vi "WASDDRIVE.vi"(9 "RIGHTIN":i8, 10 "LEFTIN":i8, 11 "KEY":i16) -> (2 "RIGHTOUT":i8, 3 "LEFTOUT":i8)   [LabVIEW 2017]
panel:
  # "This is the WASD motor control VI. It takes in key presses and outputs motor values based on those."
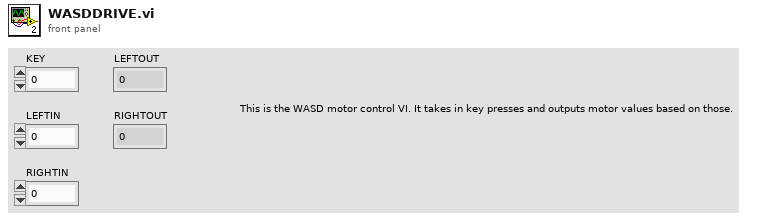
[diagram p1: front panel]
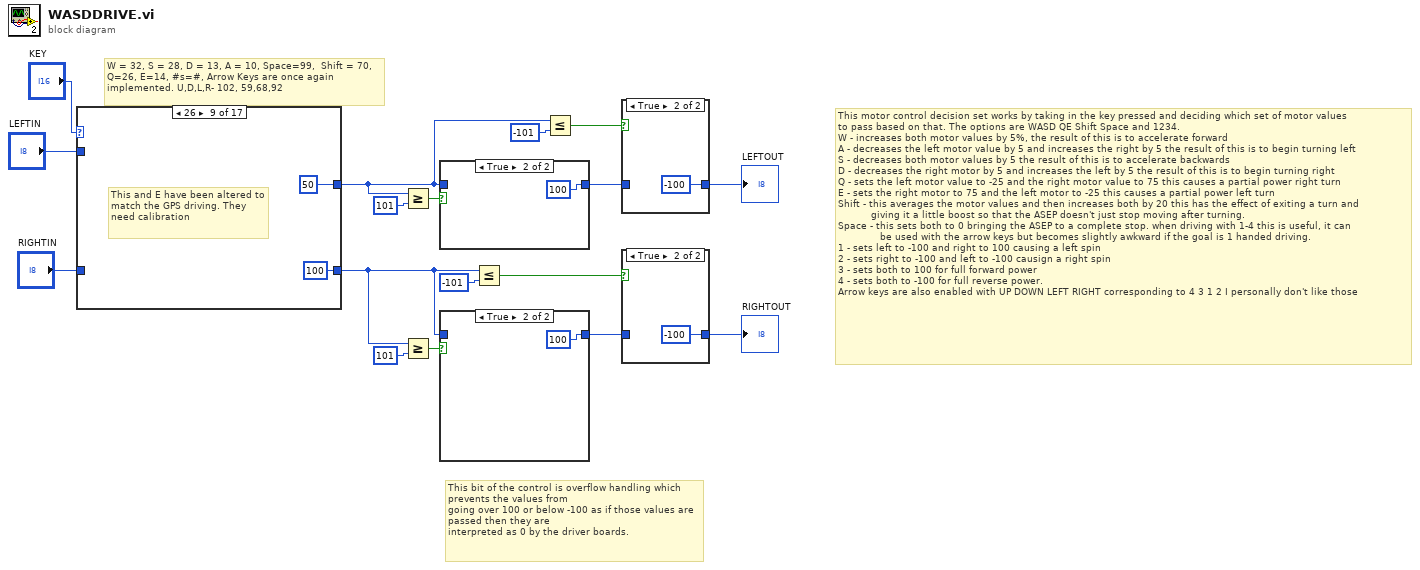
[diagram p0: block diagram]
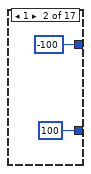
[diagram p7: hidden frame]
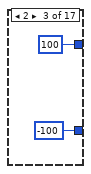
[diagram p8: hidden frame]
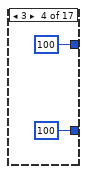
[diagram p9: hidden frame]
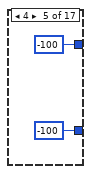
[diagram p10: hidden frame]
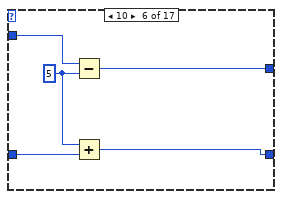
[diagram p11: hidden frame]
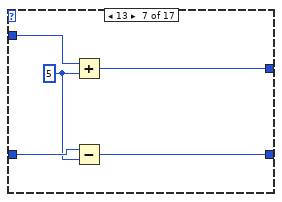
[diagram p12: hidden frame]
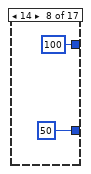
[diagram p13: hidden frame]
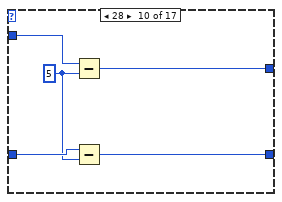
[diagram p14: hidden frame]
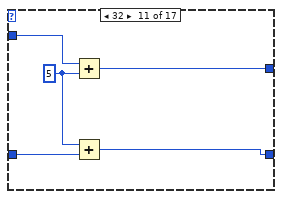
[diagram p15: hidden frame]
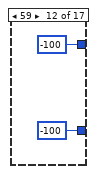
[diagram p16: hidden frame]
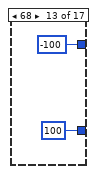
[diagram p17: hidden frame]
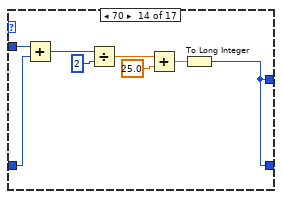
[diagram p18: hidden frame]
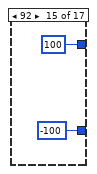
[diagram p19: hidden frame]
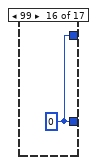
[diagram p20: hidden frame]
diagram:
  # "This bit of the control is overflow handling which prevents the values from \ngoing over 100 or below -100 as if those values are passed then they are \ninterpreted as 0 by the driver boards."
  # "This motor control decision set works by taking in the key pressed and deciding which set of motor values\nto pass based on that. The options are WASD QE Shift Space and 1234. \nW - increases both motor values by 5%, the result of this is to accelerate forward\nA - decreases the left motor value by 5 and increases the right by 5 the result of this is to begin turning left\nS - decreases both motor values by 5 the result of this is to accelerate backwards\nD - decreases the right motor by 5 and increases the left by 5 the result of this is to begin turning right\nQ - sets the left motor value to -25 and the right motor value to 75 this causes a partial power right turn\nE - sets the right motor to 75 and the left motor to -25 this causes a partial power left turn\nShift - this averages the motor values and then increases both by 20 this has the effect of exiting a turn and\n           giving it a little boost so that the ASEP doesn't just stop moving after turning. \nSpace - this sets both to 0 bringing the ASEP to a complete stop. when driving with 1-4 this is useful, it can \n              be used with the arrow keys but becomes slightly awkward if the goal is 1 handed driving. \n1 - sets left to -100 and right to 100 causing a left spin\n2 - sets right to -100 and left to -100 causign a right spin\n3 - sets both to 100 for full forward power\n4 - sets both to -100 for full reverse power.\nArrow keys are also enabled with UP DOWN LEFT RIGHT corresponding to 4 3 1 2 I personally don't like those"
  # "W = 32, S = 28, D = 13, A = 10, Space=99,  Shift = 70, Q=26, E=14, #s=#, Arrow Keys are once again implemented. U,D,L,R- 102, 59,68,92"
  n1 = case shown="26" "KEY" {
    tunnel: [w18 100 -100 100 -100 w31 w33 50 100 w43 w48 -100 100 w59 -100 w66 100] -> w14
    tunnel: [w19 -100 100 100 -100 w28 w36 100 50 w45 w47 -100 -100 w59 100 w66 100] -> w7
    tunnel: "LEFTIN" -> [w19 _ _ _ _ w29 w37 _ _ w46 w51 _ _ w63 _ _ _]
    tunnel: "RIGHTIN" -> [w18 _ _ _ _ w32 w35 _ _ w44 w49 _ _ w62 _ _ _]
    frame 0, Default {
    }
    frame 1 {
    }
    frame 2 {
    }
    frame 3 {
    }
    frame 4 {
    }
    frame 10 {
      w30 = 5
      n2 = Subtract(x=w29, y=w30) -> (x-y=w28:i32)
      n3 = Add(x=w30, y=w32) -> (x+y=w31:i32)
    }
    frame 13 {
      w34 = 5
      n4 = Add(x=w37, y=w34) -> (x+y=w36:i32)
      n5 = Subtract(x=w35, y=w34) -> (x-y=w33:i32)
    }
    frame 14 {
    }
    frame 26 {
      # "This and E have been altered to match the GPS driving. They need calibration"
    }
    frame 28 {
      w42 = 5
      n6 = Subtract(x=w46, y=w42) -> (x-y=w45:i32)
      n7 = Subtract(x=w44, y=w42) -> (x-y=w43:i32)
    }
    frame 32 {
      w50 = 5
      n8 = Add(x=w51, y=w50) -> (x+y=w47:i32)
      n9 = Add(x=w50, y=w49) -> (x+y=w48:i32)
    }
    frame 59 {
    }
    frame 68 {
    }
    frame 70 {
      n10 = Add(x=w63, y=w62) -> (x+y=w61:i8)
      n11 = Divide(x=w61, y=2) -> (x/y=w58:dbl)
      n12 = Add(x=w58, y=25.0) -> (x+y=w57:dbl)
      n13 = To Long Integer(number=w57) -> (32bit integer=w59:i32)
    }
    frame 92 {
    }
    frame 99 {
      w66 = 0
    }
    frame 102 {
    }
  }
  n14 = Greater Or Equal?(x=w7, y=101) -> (x >= y?=w6:bool)
  n15 = Greater Or Equal?(x=w14, y=101) -> (x >= y?=w13:bool)
  n16 = case shown="True" w6 {
    tunnel: [w69 100 ("y")] -> w8
    tunnel: w7 -> [w69 _]
    frame False {
    }
    frame True {
    }
  }
  n17 = case shown="True" w13 {
    tunnel: [w71 100 ("y")] -> w15
    tunnel: w14 -> [w71 _]
    frame False {
    }
    frame True {
    }
  }
  n18 = Less Or Equal?(x=w14, y=-101) -> (x <= y?=w12:bool)
  n19 = Less Or Equal?(x=w7, y=-101) -> (x <= y?=w9:bool)
  n20 = case shown="True" w9 {
    tunnel: [w73 -100 ("y")] -> w16
    tunnel: w8 -> [w73 _]
    frame False {
    }
    frame True {
    }
  }
  "LEFTOUT" <- w16
  n21 = case shown="True" w12 {
    tunnel: [w75 -100 ("y")] -> w17
    tunnel: w15 -> [w75 _]
    frame False {
    }
    frame True {
    }
  }
  "RIGHTOUT" <- w17
